vi "Build.vi"   [LabVIEW 2018, in "Scripts.lvlib"]
uses:
  Scripts.lvlib
  <vilib>/Field R&D Services/Labricator/Toolkit/Labricator.lvlib
panel:
  # "Overview: Builds all Source Distribution specifications for this project\nRequirements: LabVIEW\nInstructions: Run this VI.\n\nThis VI builds all of the build specifications for this project. Any version of LabVIEW that supports projects and the Application Builder API can be used."
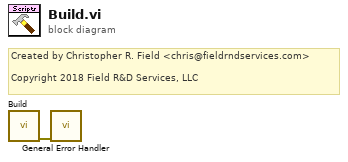
[diagram p0: block diagram]
diagram:
  # "Created by Christopher R. Field <chris@fieldrndservices.com>\n\nCopyright 2018 Field R&D Services, LLC"
  n1 = call <vilib>:"Build.vi"() -> ("Error Out"=w1:errorcluster)  [unwired: 11 in]
  n2 = call <vilib>:"General Error Handler.vi"("error in (no error)"=w1) -> ()  [unwired: 10 in, 5 out]
